vi "Build Picture path (SubVI).vi"(8 "Error In":errorcluster, 10 "Numeric in":i32, 11 "Application Directory":path) -> (0 "Error Out":errorcluster, 2 "Numeric out":i32, 3 "Path":path)   [LabVIEW 2014]
uses:
  <vilib>/MakerHub/Toolbox/LMH-Toolbox.lvlib
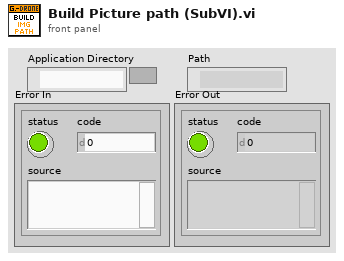
[diagram p1: front panel]
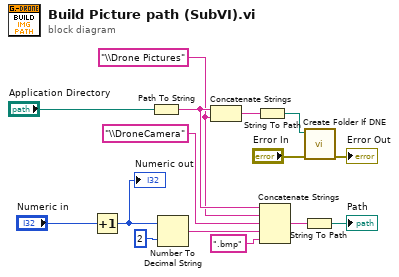
[diagram p0: block diagram]
diagram:
  w5 = "\\Drone Pictures" ("string")
  n1 = Increment(x="Numeric in") -> (x+1=w15:i32)
  "Numeric out" <- w15
  n2 = Path To String(path="Application Directory") -> (string=w6:string)
  n3 = Number To Decimal String(number=w15, width (-)=i16 2) -> (decimal integer string=w12:string)
  n4 = Concatenate Strings(w6, w5) -> (w4:string)
  n5 = String To Path(string=w4) -> (path=w3:path)
  n6 = Concatenate Strings(w6, w5, "\\DroneCamera" ("string"), w12, ".bmp" ("string")) -> (w11:string)
  n7 = String To Path(string=w11) -> (path=→"Path":path)
  n8 = call <vilib>:"Create Folder If DNE.vi"("Error In"="Error In", "Folder Path"=w3) -> ("Error Out"=→"Error Out":errorcluster)  [unwired: 8 in, 1 out]
